vi "CH_LM Action Trigger Sequence ID.vi"(0 "Meter Index":i32, 2 "Sequence ID (0)":u32, 5 "error in (no error)":errorcluster, 7 "Timeout / ms (3000)":i32=3000, 9 "Lock Timeout / ms (1000)":i32=1000) -> (11 "Lock timed out":bool, 14 "Meter Index":i32, 19 "error out":errorcluster)   [LabVIEW 2012, in "CH_LM.lvlib"]
doc: "This command will set the sequence ID.\n\nThe sequence ID is used for data synchronization of multiple meters sharing the same trigger signal. The sequence ID will be transmitted with each measurement data record if the SEQ token is specified in the CONF:READ:SEND command . The command will be ignored if the software hold state is not active."
uses:
  CH_LM.lvlib
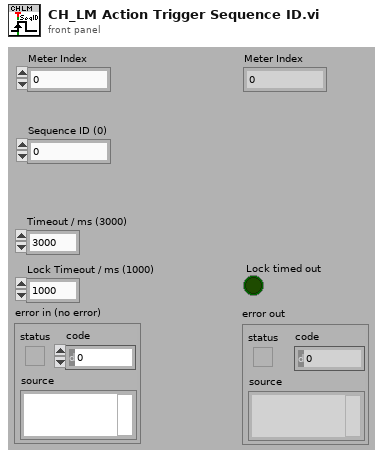
[diagram p1: front panel]
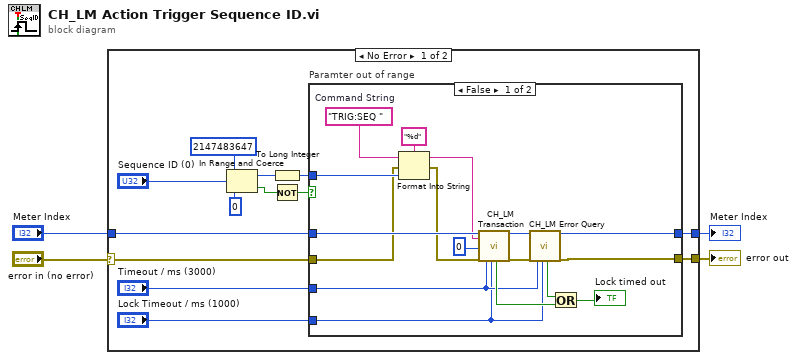
[diagram p0: block diagram]
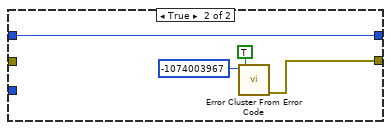
[diagram p2: hidden frame]
diagram:
  n1 = case shown="No Error" "error in (no error)" {
    selector: "error in (no error)" -> [w17 w40]
    tunnel: [w15 w40] -> w4
    tunnel: "Meter Index" -> [w16 w39]
    tunnel: [w14 w39] -> w1
    frame No Error {
      n2 = In Range and Coerce(upper limit=u32 2147483647, x="Sequence ID (0)", lower limit=u32 0) -> (coerced(x)=w11:u32, In Range?=w5:bool)
      n3 = To Long Integer(number=w11) -> (32bit integer=w8:i32)
      n4 = Not(x=w5) -> (.not. x?=w6:bool)
      n5 = case "Paramter out of range" shown="False" w6 {
        tunnel: w17 -> [w24 _]
        tunnel: w16 -> [w34 w38]
        tunnel: [w20 w36] -> w15
        tunnel: [w21 w38] -> w14
        tunnel: "Timeout / ms (3000)" -> [w27 _]
        tunnel: "Lock Timeout / ms (1000)" -> [w26 _]
        tunnel: w8 -> [w25 _]
        frame False {
          w19 = "TRIG:SEQ "  # Command String
          n6 = Format Into String(format string="%d", initial string=w19, error in=w24, w25) -> (resulting string=w18:string, error out=w23:errorcluster)
          n7 = call "CH_LM Transaction.vi"("Meter Index"=w34, "Command String"=w18, "NofStrings (-1:all)"=0 ("t"), "error in (no error)"=w23, "Timeout / ms (3000)"=w27, "Lock Timeout / ms (1000)"=w26) -> ("Lock timed out"=w29:bool, "Meter Index"=w32:i32, "error out"=w31:errorcluster)  [unwired: 11 out]
          n8 = call "CH_LM Error Query.vi"("Meter Index"=w32, "error in (no error)"=w31, "Timeout / ms (3000)"=w27, "Lock Timeout / ms (1000)"=w26) -> ("Lock timed out"=w30:bool, "Meter Index"=w21:i32, "error out"=w20:errorcluster)  [unwired: 13 out]
          n9 = Or(x=w30, y=w29) -> (x .or. y?=→"Lock timed out":bool)
        }
        frame True {
          n10 = call <vilib>:"Error Cluster From Error Code.vi"("show call chain? (False)"=TRUE, "error code (0)"=-1074003967) -> ("error out"=w36:errorcluster)  [unwired: 1 in, 6 out]
        }
      }
    }
    frame Error {
    }
  }
  "error out" <- w4
  "Meter Index" <- w1
